vi "UE9 Stream Example with EI1050.vi"() -> ()   [LabVIEW 2021]
panel:
  in  "Simulated Processing Delay [ms]":u32
  out "UD Backlog [%]":dbl format="%.2f"
  in  "AIN Range":u16(ring) items=["LJ_rgBIP5V", "LJ_rgUNI5V", "LJ_rgUNI2P5V", "LJ_rgUNI1P25V", "LJ_rgUNIP625V"]
  in  "Scan List":u8[](array[numeric])=[0, 1, 2, 3]
  out "Actual Scan Rate (Hz)":dbl=1000.0 format="%.3f"
  out "ms Per Loop":u32
  out "Comm Backlog [%]":dbl format="%.2f"
  out "Scans Retrieved Sec (measured)":dbl format="%.2f"
  out "# Scans Read":i32
  out "# of iterations":i32
  out "Data":dbl[][](array[numeric]) format="%.3f"
  in  "Scan Rate (Hz)":dbl=1000.0 format="%.3f"
  in  "Data File Extension":string="dat"
  out "Current Data File":path
  in  "Data File Prefix":string="data"
  in  "Write To File":bool
  in  "FirstFound":bool=TRUE
  in  "stop":bool
  in  "ConnectionType":u16(ring) items=["LJ_ctUSB", "LJ_ctETHERNET"]
  in  "DeviceType":u16(ring)=1 items=["LJ_dtU3", "LJ_dtUE9"]
  in  "Address":string="192.168.1.209"
  out "Error Message":string
  in  "Resolution":i32=12
  # "The actual scans/sec is controlled\nby hardware and is known.  This\n\"measured\" suggests the rate at\nwhich data is being retreived."
  # "Specify an IP address for Ethernet, or Local ID\nfor USB.  If FirstFound is selected, Local ID is\nignored for USB.  Clear FirstFound if using Ethernet."
  # "(for all channels)"
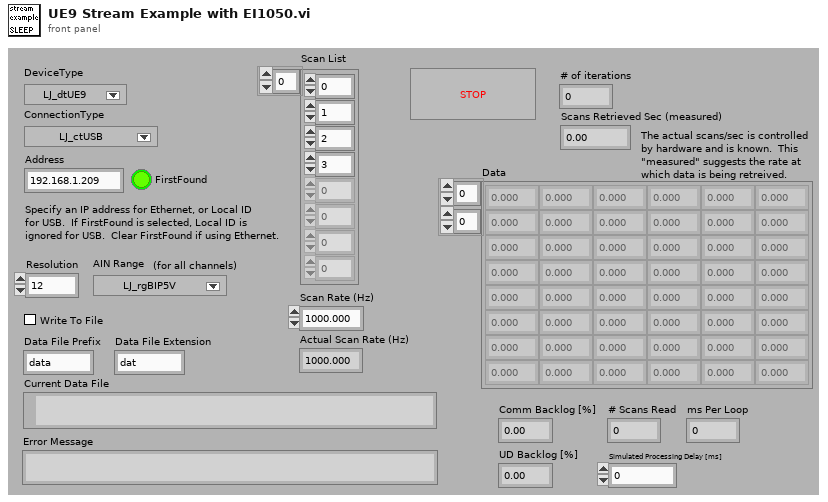
[diagram p1: front panel]
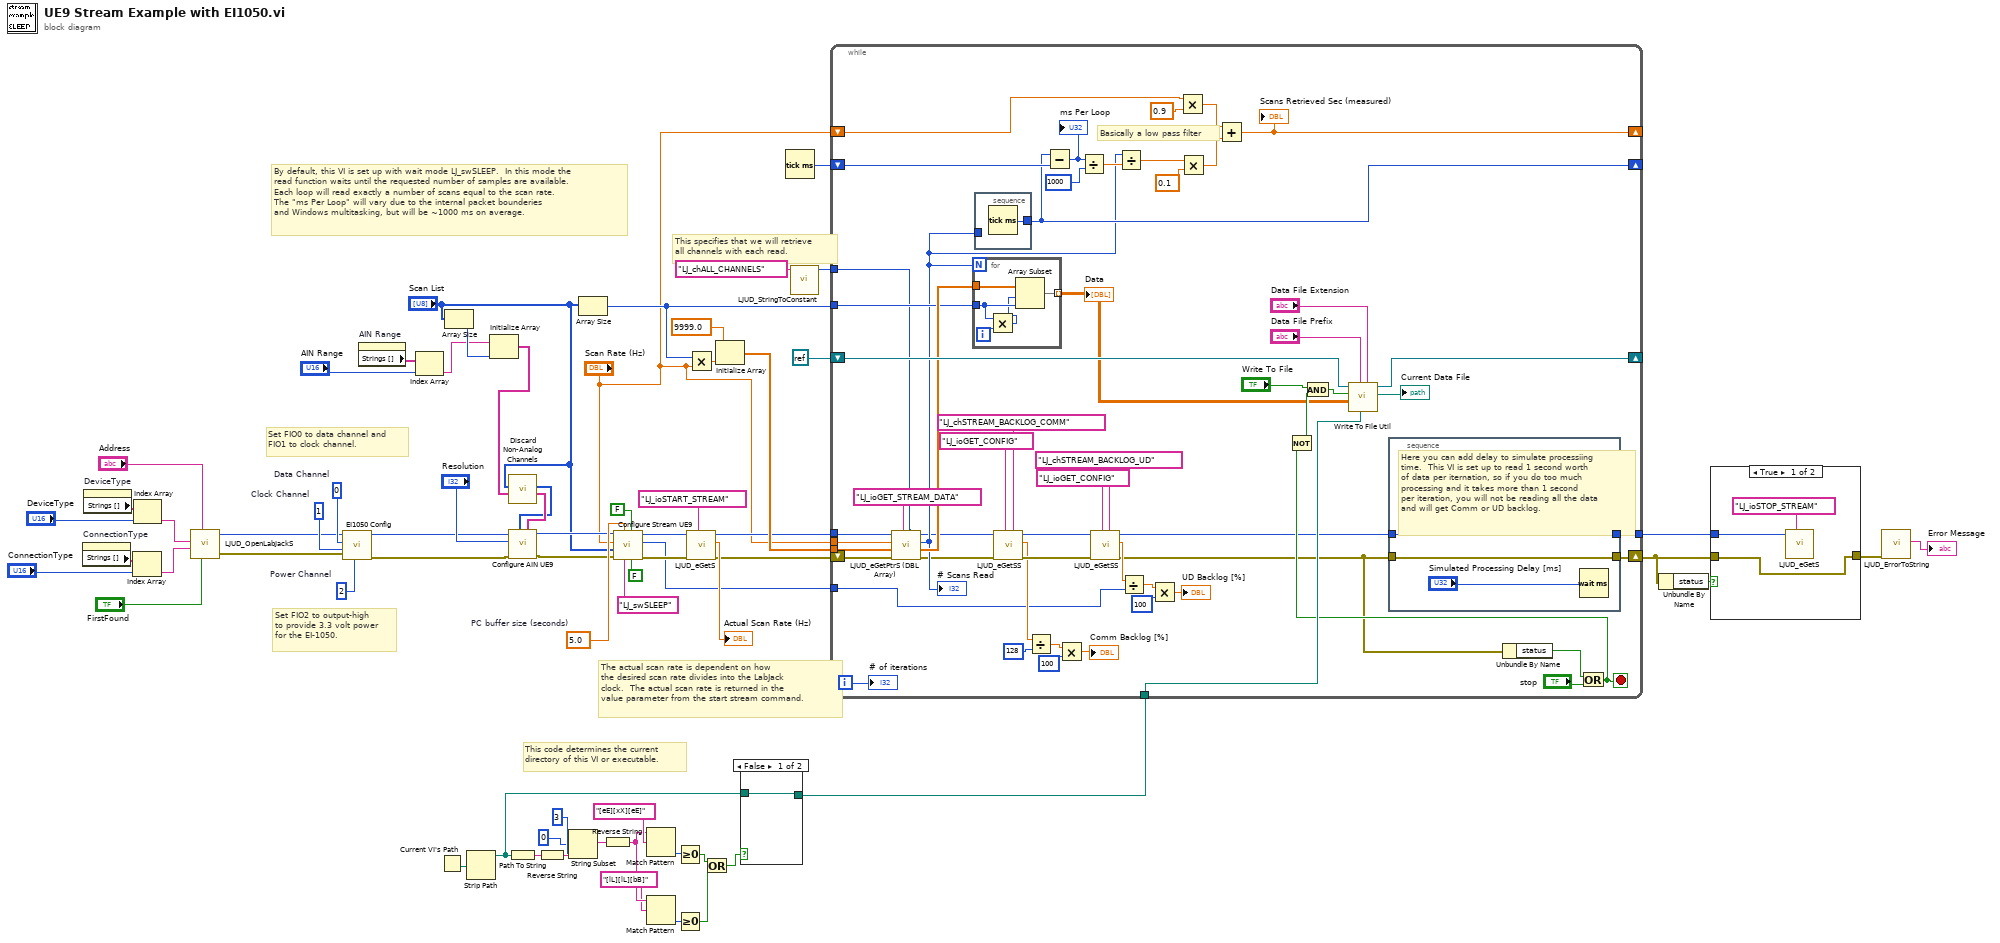
[diagram p0: block diagram]
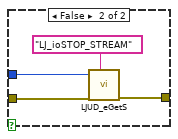
[diagram p2: hidden frame]
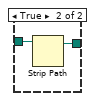
[diagram p3: hidden frame]
diagram:
  w5 = 0  # Data Channel
  w6 = 1  # Clock Channel
  w7 = 2  # Power Channel
  w36 = 5.0  # PC buffer size (seconds)
  # "Set FIO0 to data channel and\nFIO1 to clock channel."
  # "Set FIO2 to output-high\nto provide 3.3 volt power\nfor the EI-1050."
  # "This specifies that we will retrieve\nall channels with each read."
  # "The actual scan rate is dependent on how\nthe desired scan rate divides into the LabJack\nclock.  The actual scan rate is returned in the\nvalue parameter from the start stream command."
  # "By default, this VI is set up with wait mode LJ_swSLEEP.  In this mode the\nread function waits until the requested number of samples are available.\nEach loop will read exactly a number of scans equal to the scan rate.\nThe \"ms Per Loop\" will vary due to the internal packet bounderies\nand Windows multitasking, but will be ~1000 ms on average."
  # "This code determines the current\ndirectory of this VI or executable."
  n1 = property on="ConnectionType" class="Ring (strict)"() -> ("Strings []"=w22:string[])  [unwired: 2 in, 2 out]
  n2 = property on="DeviceType" class="Ring (strict)"() -> ("Strings []"=w23:string[])  [unwired: 2 in, 2 out]
  n3 = Index Array(array=w22, index="ConnectionType") -> (element=w18:string)
  n4 = Index Array(array=w23, index="DeviceType") -> (element=w19:string)
  n5 = call "LJUD_OpenLabJackS.vi"("FirstFound"="FirstFound", "Address"="Address", "ConnectionType"=w18, "DeviceType"=w19) -> ("error out"=w4:errorcluster, "Handle"=w1:i32)  [unwired: 5 in, 1 out]
  n6 = call "EI1050 Config.vi"("Power Channel"=w7, "error in"=w4, "Clock Channel"=w6, "Data Channel"=w5, "Handle In"=w1) -> ("error out"=w2:errorcluster, "Handle Out"=w3:i32)  [unwired: 5 in]
  n7 = property on="AIN Range" class="Ring (strict)"() -> ("Strings []"=w25:string[])  [unwired: 2 in, 2 out]
  n8 = Index Array(array=w25, index="AIN Range") -> (element=w26:string)
  n9 = Current VI's Path() -> (path=w64:path)
  n10 = Array Size(array="Scan List") -> (size(s)=w29:i32)
  n11 = Strip Path(path=w64) -> (stripped path=w56:path)  [unwired: 1 out]
  n12 = Initialize Array(w26, w29) -> (w14:string[])
  n13 = call "Discard Non-Analog Channels.vi"("Ranges In"=w14, "Channels In"="Scan List") -> ("Ranges Out"=w12:string[], "Channels Out"=w11:i32[])  [unwired: 6 in, 2 out]
  n14 = call "Configure AIN UE9.vi"("Ranges"=w12, "Channels"=w11, "error in"=w2, "Resolution"="Resolution", "Handle In"=w3) -> ("error out"=w32:errorcluster, "Handle Out"=w31:i32)  [unwired: 5 in]
  n15 = Path To String(path=w56) -> (string=w63:string)
  n16 = Reverse String(1:w63) -> (0:w62:string)
  n17 = String Subset(string=w62, offset (0)=0, length (rest)=3 ("length")) -> (substring=w59:string)
  n18 = Array Size(array="Scan List") -> (size(s)=w42:i32)
  n19 = Reverse String(1:w59) -> (0:w55:string)
  n20 = call "Configure Stream UE9.vi"("External Scan Trigger"=FALSE, "Scan Clock Output"=FALSE, "Wait Mode"="LJ_swSLEEP" ("Wait Mode (2)"), "PC buffer size (seconds)"=w36, "error in"=w32, "Scan List"="Scan List", "Scan Rate (Hz)"="Scan Rate (Hz)", "Handle In"=w31) -> ("error out"=w46:errorcluster, "PC buffer size (samples)"=w8:i32, "Handle Out"=w47:i32)  [unwired: 1 in]
  n21 = Match Pattern(string=w55, regular expression="[eE][xX][eE]") -> (offset past match=w57:i32)  [unwired: 1 in, 3 out]
  n22 = Match Pattern(string=w55, regular expression="[lL][lL][bB]") -> (offset past match=w52:i32)  [unwired: 1 in, 3 out]
  n23 = Greater Or Equal To 0?(x=w57) -> (x >= 0?=w53:bool)
  n24 = Greater Or Equal To 0?(x=w52) -> (x >= 0?=w51:bool)
  n25 = Multiply(x=w42, y="Scan Rate (Hz)") -> (x*y=w45:dbl)
  n26 = call "LJUD_eGetS.vi"("IOType"="LJ_ioSTART_STREAM", "error in"=w46, "Handle In"=w47) -> ("error out"=w10:errorcluster, "Value Read"=→"Actual Scan Rate (Hz)":dbl, "Handle Out"=w28:i32)  [unwired: 6 in]
  n27 = Or(x=w53, y=w51) -> (x .or. y?=w50:bool)
  n28 = Initialize Array(9999.0, w45) -> (w43:dbl[])
  n29 = case shown="False" w50 {
    tunnel: w56 -> [w68 w70]
    tunnel: [w68 w69] -> w49
    frame False {
    }
    frame True {
      n30 = Strip Path(path=w70) -> (stripped path=w69:path)  [unwired: 1 out]
    }
  }
  n31 = Tick Count (ms)() -> (millisecond timer value=w37:u32)
  n32 = call "LJUD_StringToConstant.vi"("String"="LJ_chALL_CHANNELS") -> ("Constant Number"=w15:i32)  [unwired: 9 in, 1 out]
  n33 = while {
    tunnel: w8 -> [w77]
    shift-left: w10 -> [w85]
    shift-right: [w73] -> w9
    tunnel: w15 -> [w90]
    shift-left: "Scan Rate (Hz)" -> [w99]
    shift-right: [w96] -> _
    shift-left: w37 -> [w108]
    shift-right: [w105] -> _
    tunnel: [w71] -> w40
    tunnel: w42 -> [w110]
    tunnel: w43 -> [w113]
    tunnel: "Scan Rate (Hz)" -> [w111]
    tunnel: w49 -> [w117]
    shift-left: refnum<k0> refnum -> [w123]
    shift-right: [w122] -> _
    tunnel: w28 -> [w115]
    i -> [w109]
    stop <- w116 stop-if-true
    # "Basically a low pass filter"
    n34 = call "LJUD_eGetPtrS (DBL Array).vi"("Channel"=w90, "IOType"="LJ_ioGET_STREAM_DATA", "error in"=w85, "DBL Array Write"=w113, "Value"=w111, "Handle In"=w115) -> ("error out"=w94:errorcluster, "DBL Array Read"=w112:dbl[], "Value"=w103:i32, "Handle Out"=w95:i32)  [unwired: 2 in]
    "# Scans Read" <- w103
    n35 = for {
      N: w103 -> [_]
      tunnel: w112 -> [w136]
      tunnel: w110 -> [w135]
      tunnel: [w132] -> w91 mode=indexing
      i -> [w134]
      n36 = Multiply(x=w135, y=w134) -> (x*y=w133:i32)
      n37 = Array Subset(array=w136, index=w133, length=w135) -> (w132:dbl[])
    }
    "Data" <- w91
    n38 = stacked-sequence {
      tunnel: w103 -> [_]
      tunnel: [w131] -> w105
      frame #0 {
        n39 = Tick Count (ms)() -> (millisecond timer value=w131:u32)
      }
    }
    n40 = call "LJUD_eGetSS.vi"("Channel"="LJ_chSTREAM_BACKLOG_COMM", "IOType"="LJ_ioGET_CONFIG", "error in"=w94, "Handle In"=w95) -> ("error out"=w86:errorcluster, "Value Read"=w81:dbl, "Handle Out"=w87:i32)  [unwired: 5 in]
    n41 = Divide(x=w81, y=128) -> (x/y=w84:dbl)
    n42 = Subtract(x=w105, y=w108) -> (x-y=w107:u32)
    "ms Per Loop" <- w107
    n43 = Multiply(x=w84, y=100) -> (x*y=→"Comm Backlog [%]":dbl)
    n44 = Divide(x=w107, y=u32 1000) -> (x/y=w104:dbl)
    n45 = call "LJUD_eGetSS.vi"("Channel"="LJ_chSTREAM_BACKLOG_UD", "IOType"="LJ_ioGET_CONFIG", "error in"=w86, "Handle In"=w87) -> ("error out"=w74:errorcluster, "Value Read"=w76:dbl, "Handle Out"=w72:i32)  [unwired: 5 in]
    n46 = Divide(x=w103, y=w104) -> (x/y=w102:dbl)
    n47 = Divide(x=w76, y=w77) -> (x/y=w78:dbl)
    n48 = Multiply(x=w78, y=100) -> (x*y=→"UD Backlog [%]":dbl)
    n49 = Multiply(x=w99, y=0.9) -> (x*y=w98:dbl)
    n50 = Multiply(x=w102, y=0.1) -> (x*y=w97:dbl)
    n51 = Add(x=w98, y=w97) -> (x+y=w96:dbl)
    "Scans Retrieved Sec (measured)" <- w96
    n52 = stacked-sequence {
      tunnel: w74 -> [w130]
      tunnel: [w130] -> w73
      tunnel: w72 -> [w129]
      tunnel: [w129] -> w71
      frame #0 {
        # "Here you can add delay to simulate processiing\ntime.  This VI is set up to read 1 second worth\nof data per iternation, so if you do too much\nprocessing and it takes more than 1 second\nper iteration, you will not be reading all the data\nand will get Comm or UD backlog."
        n53 = Wait (ms)(milliseconds to wait="Simulated Processing Delay [ms]") -> ()  [unwired: 1 out]
      }
    }
    n54 = Unbundle By Name(w74) -> ("status"=w126:bool)
    n55 = Or(x=w126, y="stop") -> (x .or. y?=w116:bool)
    n56 = Not(x=w116) -> (.not. x?=w118:bool)
    n57 = And(x="Write To File", y=w118) -> (x .and. y?=w119:bool)
    n58 = call "Write To File Util.vi"("Data File Extension"="Data File Extension", "Working Directory"=w117, "Data File Prefix"="Data File Prefix", "Data"=w91, "Write To File"=w119, "File Refnum In"=w123) -> ("Current Data File"=→"Current Data File":path, "File Refnum Out"=w122:refnum<file>)  [unwired: 3 in, 1 out]
    "# of iterations" <- w109
  }
  n59 = Unbundle By Name(w9) -> ("status"=w17:bool)
  n60 = case shown="True" w17 {
    tunnel: w40 -> [w138 w142]
    tunnel: [w137 w141] -> w39
    tunnel: w9 -> [w137 w140]
    frame True {
      n61 = call "LJUD_eGetS.vi"("IOType"="LJ_ioSTOP_STREAM", "Handle In"=w138) -> ()  [unwired: 7 in, 3 out]
    }
    frame False {
      n62 = call "LJUD_eGetS.vi"("IOType"="LJ_ioSTOP_STREAM", "error in"=w140, "Handle In"=w142) -> ("error out"=w141:errorcluster)  [unwired: 6 in, 2 out]
    }
  }
  n63 = call "LJUD_ErrorToString.vi"("error in"=w39) -> ("String"=→"Error Message":string)  [unwired: 10 in]
